vi "Cursors4Contrast_v2.vi"(3 "Cursor 2":dbl, 4 "Cursor 1":dbl, 5 "Spectres vs PZA":dbl[][](array[numeric]), 6 "Energy":dbl[](array[numeric])) -> (0 "Contrast of ROI vs PZC":dbl[](array[numeric]), 1 "Spectra ROI":dbl[][](array[numeric]), 2 "Energy ROI":dbl[](array[numeric]))   [LabVIEW 2019]
panel:
  out "size(s)":i32
  # "(dim: Nx1380)"
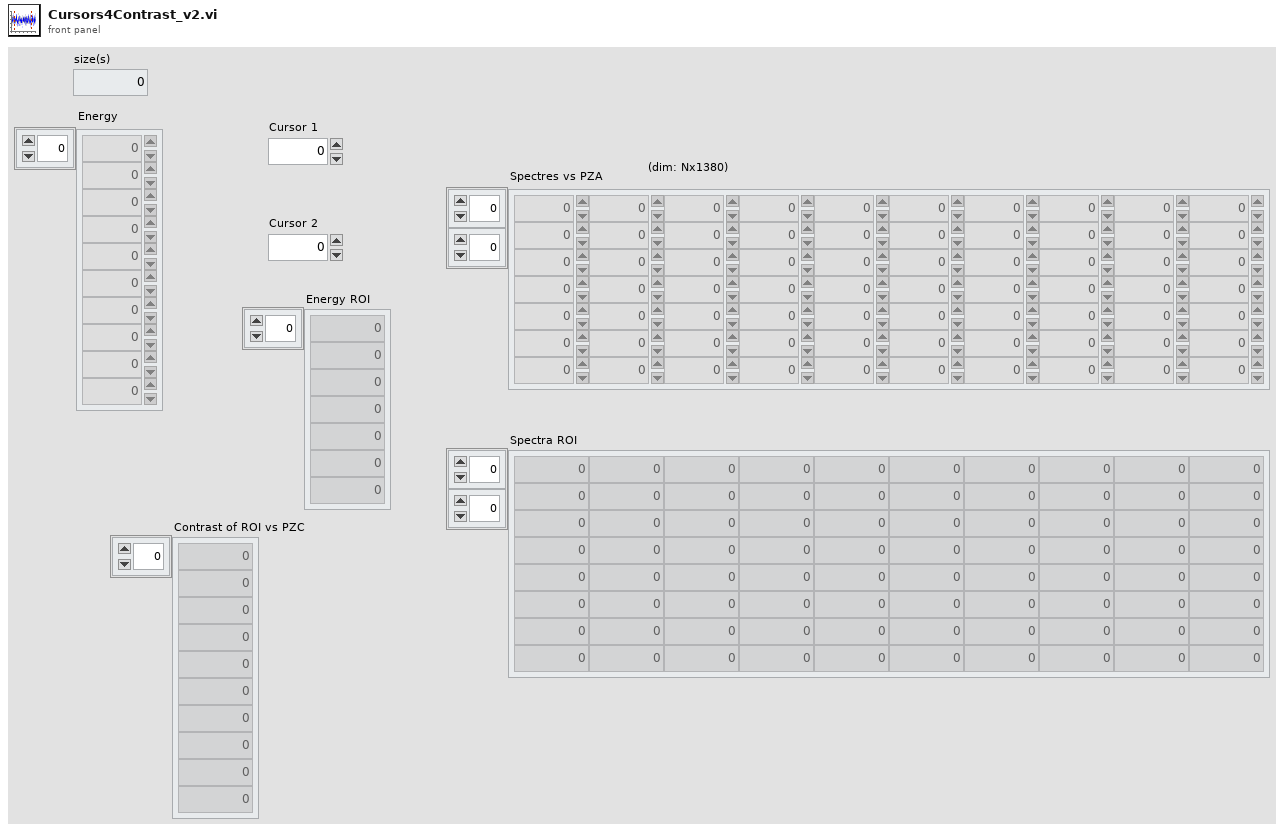
[diagram p1: front panel]
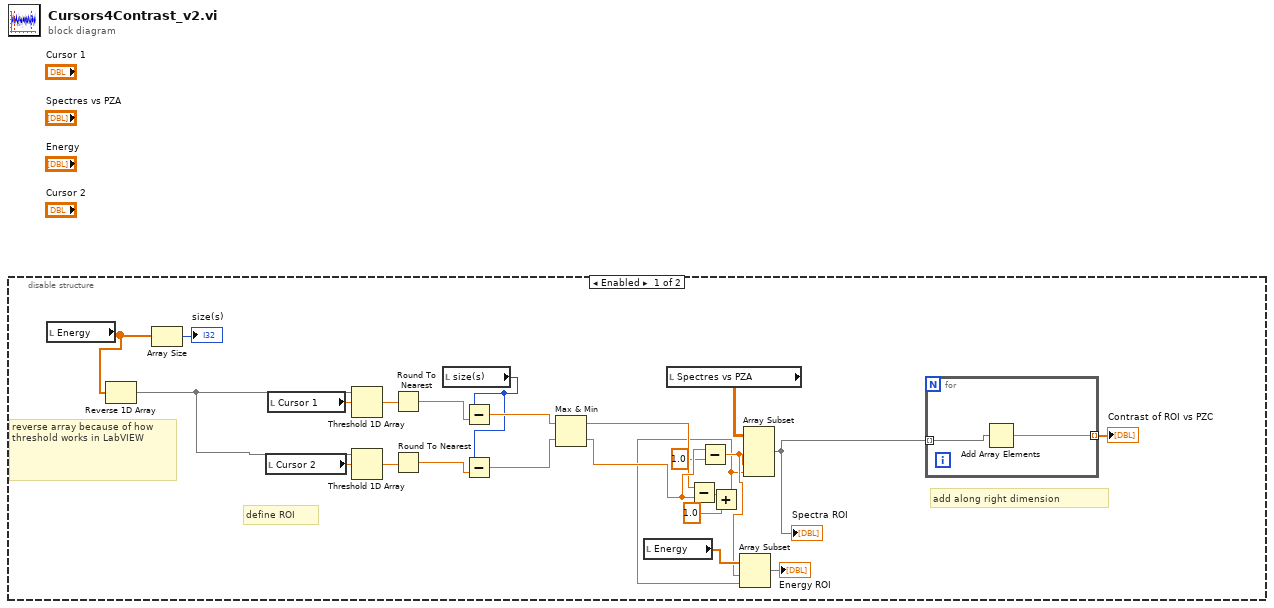
[diagram p0: block diagram]
diagram:
  n1 = disable-structure shown="Enabled" {
    frame Enabled {
      # "add along right dimension"
      # "reverse array because of how threshold works in LabVIEW"
      # "define ROI"
      n2 = local read "Energy"() -> (w15:dbl[])
      n3 = Reverse 1D Array(array=w15) -> (reversed array=w24:dbl[])
      n4 = Array Size(array=w15) -> (size(s)=→"size(s)":i32)
      n5 = local read "Cursor 2"() -> (w13:dbl)
      n6 = local read "Cursor 1"() -> (w14:dbl)
      n7 = Threshold 1D Array(2:w14, 3:w24) -> (0:w12:dbl)  [unwired: 1 in]
      n8 = Threshold 1D Array(2:w13, 3:w24) -> (0:w11:dbl)  [unwired: 1 in]
      n9 = Round To Nearest(number=w12) -> (nearest integer value=w23:dbl)
      n10 = Round To Nearest(number=w11) -> (nearest integer value=w22:dbl)
      n11 = local read "size(s)"() -> (w10:i32)
      n12 = Subtract(x=w10, y=w23) -> (x-y=w21:dbl)
      n13 = Subtract(x=w10, y=w22) -> (x-y=w20:dbl)
      n14 = Max & Min(x=w21, y=w20) -> (max(x,y)=w18:dbl, min(x,y)=w19:dbl)
      n15 = local read "Energy"() -> (w4:dbl[])
      n16 = local read "Spectres vs PZA"() -> (w9:dbl[][])
      n17 = Subtract(x=w18, y=w19) -> (x-y=w6:dbl)
      n18 = Subtract(x=w19, y=1.0) -> (x-y=w3:dbl)
      n19 = Add(x=w6, y=1.0) -> (x+y=w2:dbl)
      n20 = Array Subset(array=w4, index=w3, length=w2) -> (→"Energy ROI":dbl[])
      n21 = Array Subset(array=w9, index (col)=w3, length (col)=w2) -> (w17:dbl[][])  [unwired: 2 in]
      "Spectra ROI" <- w17
      n22 = for {
        tunnel: w17 -> [w26] mode=indexing
        tunnel: [w25] -> w5 mode=indexing
        n23 = Add Array Elements(numeric array=w26) -> (sum=w25:dbl)
      }
      "Contrast of ROI vs PZC" <- w5
    }
    frame Disabled {
    }
  }
